vi "F Dwf Analog Out Play Status.vi"(0 "hdwf":i32, 1 "cdDataCorrupted":i32, 5 "idxChannel":i32, 7 "cdDataFree":i32, 9 "cdDataLost":i32, 11 "error in (no error)":errorcluster) -> (3 "cdDataCorrupted out":i32, 4 "function return":i32, 8 "cdDataFree out":i32, 10 "cdDataLost out":i32, 15 "error out":errorcluster)   [LabVIEW 2019, in "Olasdwf.lvlib"]
doc: "DWFAPI int FDwfAnalogOutPlayStatus(HDWF hdwf, int idxChannel, int *cdDataFree, int *cdDataLost, int *cdDataCorrupted);"
uses:
  Olasdwf.lvlib
  Windows/System32/dwf.dll
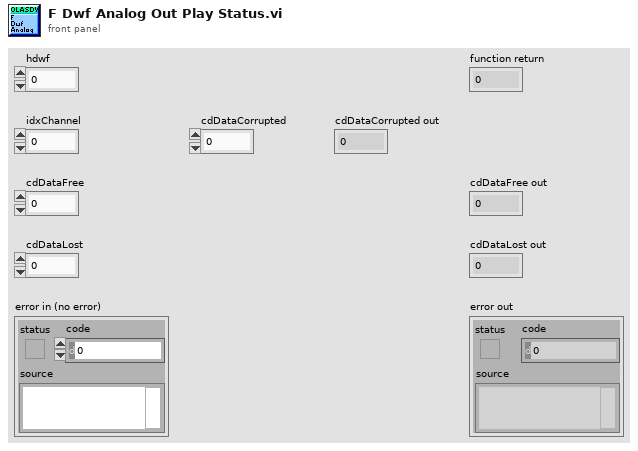
[diagram p1: front panel]
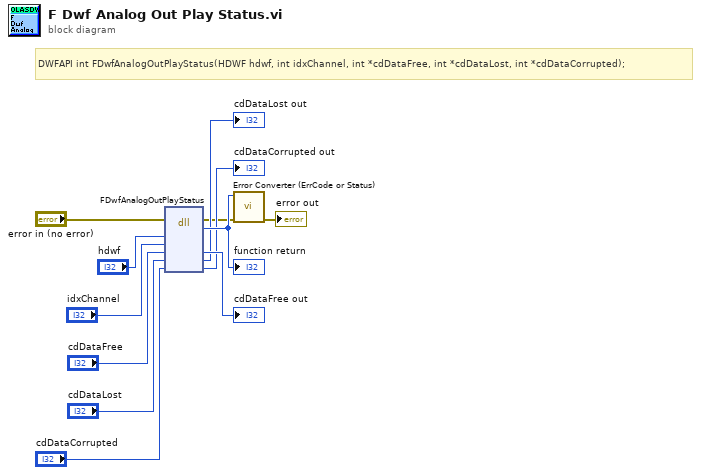
[diagram p0: block diagram]
diagram:
  # "DWFAPI int FDwfAnalogOutPlayStatus(HDWF hdwf, int idxChannel, int *cdDataFree, int *cdDataLost, int *cdDataCorrupted);"
  n1 = dll-call lib="C:/Windows/System32/dwf.*" fn="FDwfAnalogOutPlayStatus"(error in="error in (no error)", "hdwf"="hdwf", "idxChannel"="idxChannel", "cdDataFree"="cdDataFree", "cdDataLost"="cdDataLost", "cdDataCorrupted"="cdDataCorrupted") -> (error out=w2:errorcluster, w12:i32, "cdDataFree"=→"cdDataFree out":i32, "cdDataLost"=→"cdDataLost out":i32, "cdDataCorrupted"=→"cdDataCorrupted out":i32)  [unwired: 4 in, 1 out]
  "function return" <- w12
  n2 = call "Error Converter (ErrCode or Status).vi"("error in (no error)"=w2, "error code"=w12) -> ("error out"=→"error out":errorcluster)  [unwired: 9 in]
